vi "LEBITplc.PubListOfBases.vi"(0 "i ref in":refnum<vi>, 2 "i attribute in":T1, 5 "error in":errorcluster) -> (14 "i ref out":refnum<vi>, 16 "i attribute out":T1, 17 "List of Bases serviceID":i32, 19 "error out":errorcluster)   [LabVIEW 2014, in "LEBITplc.lvlib"]
uses:
  LEBITplc.lvlib
  LEBITplc.i attribute.ctl
  CSlibraries/UtilityLib/UtilityLib.valueStatus.ctl
  CSlibraries/UtilityLib/UtilityLib.lvlib
  CS_Core/CSSystem/CoreLib/CoreLib.lvlib
  CSlibraries-extern/DimLVEvent/LVDimInterface/LVDimInterface.lvlib
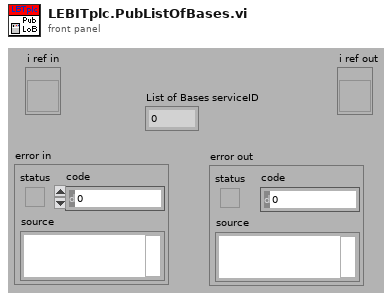
[diagram p1: front panel]
types:
  T1 = typedef "LEBITplc.lvlib/LEBITplc.i attribute.ctl" = cluster{"LLFLocation":string, "SetFileLocation":string, "nickNames":string[], "setValuePLCServiceID":i32[], "GUIServiceID":i32[], "monValuePLC":string[], "SetValueServiceID":i32[], "MonValueServiceID":i32[], "SetValue":dbl[][], "SetValueMin":dbl[], "SetValueMax":dbl[], "SetValueInfoServiceID":i32[], "GUINames":string[], "ListOfBases":string[], "Scale":dbl[], "Offset":dbl[], "setValuePLC":string[], "BaseName":string[], "ScaleServiceID":i32[], "OffsetServiceID":i32[], "AllPLCValues":string[], "CondSpecialArray":string[][], "CondSpecialIndex":i32[], "CondSpecialMonValue":dbl[], "RecentlyChanged":i32[], "SetFileLocationID":i32, "Dependent-Monitors":string[][], "LastLoadedFiles":string[], "IonGuideCalibLocation":string, "Monitor Dependent":string[], "Special":string[], "PLC?":bool[], "Start Date":string, "ListOfBasesServiceID":i32, "SETRA VISA resource":refnum<visa-resource-name>}
  T2 = typedef "UtilityLib.lvlib/UtilityLib.valueStatus.ctl" = enum16{"no info available", "stand by/off", "on", "warning", "alarm/malfunction", "not implemented", "user action required", "important information", "system default", "control default", "indicator default", "button default"}
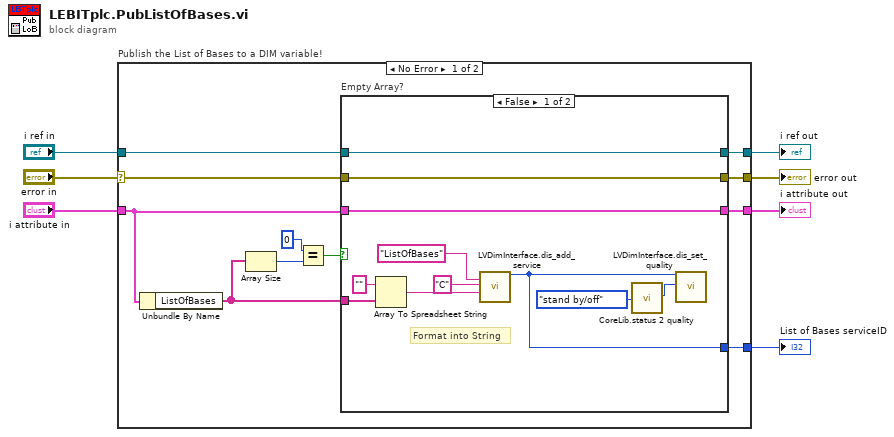
[diagram p0: block diagram]
diagram:
  n1 = case "Publish the List of Bases to a DIM variable!" shown="No Error" "error in" {
    selector: "error in" -> [w14 w34]
    tunnel: "i attribute in" -> [w13 w33]
    tunnel: [w18 w34] -> w6
    tunnel: [w17 w35] -> w5
    tunnel: "i ref in" -> [w16 w35]
    tunnel: [w15 _] -> w1
    tunnel: [w12 w33] -> w2
    frame No Error {
      n2 = Unbundle By Name(w13) -> ("ListOfBases"=w8:string[])
      n3 = Array Size(array=w8) -> (size(s)=w9:i32)
      n4 = Equal?(x=0, y=w9) -> (x = y?=w11:bool)
      n5 = case "Empty Array?" shown="False" w11 {
        tunnel: [w29 w31] -> w18
        tunnel: [w28 w32] -> w17
        tunnel: w16 -> [w28 w32]
        tunnel: [w23 _] -> w15
        tunnel: w14 -> [w29 w31]
        tunnel: w13 -> [w27 w30]
        tunnel: [w27 w30] -> w12
        tunnel: w8 -> [w22 _]
        frame False {
          # "Format into String"
          n6 = Array To Spreadsheet String(array=w22, 3:"" ("format string")) -> (spreadsheet string=w21:string)  [unwired: 1 in]
          n7 = call "LVDimInterface.dis_add_service.vi"("serviceName"="ListOfBases", "typeDescriptor"="C", "data"=w21) -> ("my_serviceID"=w23:i32)  [unwired: 15 in, 1 out]
          n8 = call "CoreLib.status 2 quality.vi"("valueStatus"=UtilityLib.valueStatus."stand by/off") -> ("quality"=w26:i32)  [unwired: 18 in]
          n9 = call "LVDimInterface.dis_set_quality.vi"("my_serviceID"=w23, "quality"=w26) -> ()  [unwired: 16 in, 2 out]
        }
        frame True {
        }
      }
    }
    frame Error {
    }
  }
  "error out" <- w6
  "i ref out" <- w5
  "i attribute out" <- w2
  "List of Bases serviceID" <- w1
